vi "Project Parser_Identify External Folders and Internal Relative Paths.vi"(7 "To Lower Case?(T)":bool=TRUE, 8 "error in (no error)":errorcluster, 11 "Project Files":string[](array[string])) -> (0 "error out":errorcluster, 2 "Internal Relative Paths":string[](array[string]), 3 "External Folder Combinations":string[](array[string]))   [LabVIEW 2019, in "Project.Dependencies Finder.lvlib"]
doc: "Split 'Project Files' into array of 'Internal Relative Paths' and 'External Folder Names'.\n\n2020-11-13: Henrik Dueholm Hansen"
uses:
  Project.Dependencies Finder.lvlib
  8584cef7-6435-468f-b24b-0a43cbeddf19.vi
  adfe3204-eb0e-4237-ad1b-a1e7be6d89d0.vi
  135987d9-7b10-437c-9908-5d0a6e40ecd4.vi
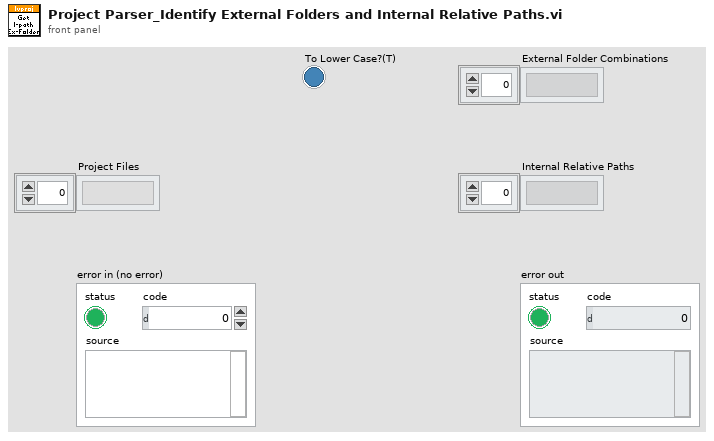
[diagram p1: front panel]
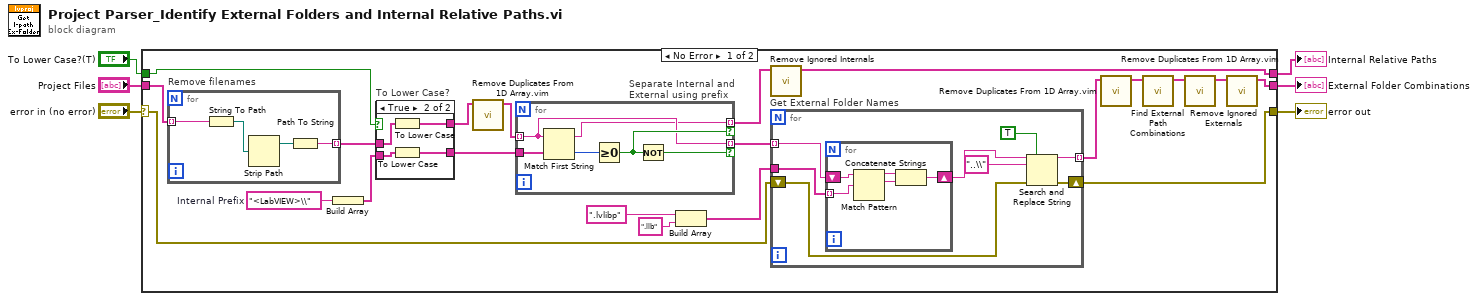
[diagram p0: block diagram]
diagram:
  n1 = case shown="No Error" "error in (no error)" {
    selector: "error in (no error)" -> [w18 w57]
    tunnel: "To Lower Case?(T)" -> [w27 _]
    tunnel: "Project Files" -> [w26 _]
    tunnel: [w12 _] -> w4
    tunnel: [w9 _] -> w3
    tunnel: [w17 w57] -> w1
    frame No Error {
      w21 = "<LabVIEW>\\"  # Internal Prefix
      n2 = for "Remove filenames" {
        tunnel: w26 -> [w56] mode=indexing
        tunnel: [w53] -> w7 mode=indexing
        n3 = String To Path(string=w56) -> (path=w55:path)
        n4 = Strip Path(path=w55) -> (stripped path=w54:path)  [unwired: 1 out]
        n5 = Path To String(path=w54) -> (string=w53:string)
      }
      n6 = Build Array(w21) -> (w20:string[])
      n7 = case "To Lower Case?" shown="True" w27 {
        tunnel: [w29 w33] -> w24
        tunnel: w20 -> [w29 w32]
        tunnel: [w28 w30] -> w8
        tunnel: w7 -> [w28 w31]
        frame False {
        }
        frame True {
          n8 = To Lower Case(string=w31) -> (all lower case string=w30:string[])
          n9 = To Lower Case(string=w32) -> (all lower case string=w33:string[])
        }
      }
      n10 = call "Remove Duplicates From 1D Array.vim"("array"=w8) -> ("array with duplicates removed"=w25:string[])  [unwired: 10 in]
      n11 = for "Separate Internal and External using prefix" {
        tunnel: w25 -> [w50] mode=indexing
        tunnel: [w47] -> w13 mode=indexing if=w51
        tunnel: [w50] -> w22 mode=indexing if=w49
        tunnel: w24 -> [w48]
        n12 = Match First String(2:w48, 3:w50) -> (0:w52:i32, 1:w47:string)
        n13 = Greater Or Equal To 0?(x=w52) -> (x >= 0?=w51:bool)
        n14 = Not(x=w51) -> (.not. x?=w49:bool)
      }
      n15 = Build Array(".lvlibp", ".llb") -> (w14:string[])
      n16 = call "Remove Ignored Internals.vi"("Internals in"=w13) -> ("Internals out"=w12:string[])  [unwired: 10 in]
      n17 = for "Get External Folder Names" {
        tunnel: w22 -> [w41] mode=indexing
        tunnel: [w34] -> w23 mode=indexing
        shift-right: [w36] -> w17
        shift-left: w18 -> [w37]
        tunnel: w14 -> [w35]
        n18 = for {
          tunnel: w35 -> [w46] mode=indexing
          shift-right: [w42] -> w40
          shift-left: w41 -> [w43]
          n19 = Match Pattern(string=w43, regular expression=w46) -> (before substring=w45:string, match substring=w44:string)  [unwired: 1 in, 2 out]
          n20 = Concatenate Strings(w45, w44) -> (w42:string)
        }
        n21 = Search and Replace String(replace all?=TRUE ("replace all? (F)"), input string=w40, search string="..\\", error in=w37) -> (result string=w34:string, error out=w36:errorcluster)  [unwired: 4 in, 2 out]
      }
      n22 = call "Remove Duplicates From 1D Array.vim"("array"=w23) -> ("array with duplicates removed"=w19:string[])  [unwired: 10 in]
      n23 = call "Find External Path Combinations.vi"("Found Common Paths in"=w19) -> ("External Path Combinations"=w10:string[])  [unwired: 10 in]
      n24 = call "Remove Duplicates From 1D Array.vim"("array"=w10) -> ("array with duplicates removed"=w11:string[])  [unwired: 10 in]
      n25 = call "Remove Ignored Externals.vi"("Externals in"=w11) -> ("Externals out"=w9:string[])  [unwired: 10 in]
    }
    frame Error {
    }
  }
  "error out" <- w1
  "Internal Relative Paths" <- w4
  "External Folder Combinations" <- w3
